vi "ueye check capture status.vi"(8 "error in (no error)":errorcluster, 11 "Camera in":refnum<k24>) -> (0 "error out":errorcluster, 2 "Error List":map{string, u64}(c390), 3 "Camera out":refnum<k24>)   [LabVIEW 2022 SP3, in "Vision.lvlib"]
uses:
  Vision.lvlib
  C:/Users/Caleb/Desktop/nebraska-silicon-lab/pixel-gantry-control/Gantry/Shared Components/bin/uEyeDotNet.dll
  bin/uEyeDotNet.dll
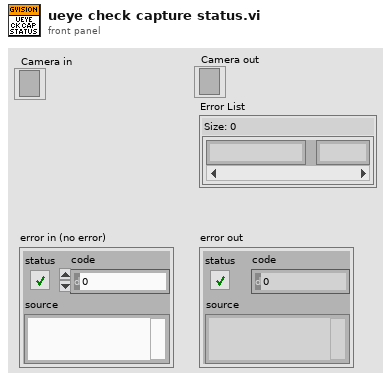
[diagram p1: front panel]
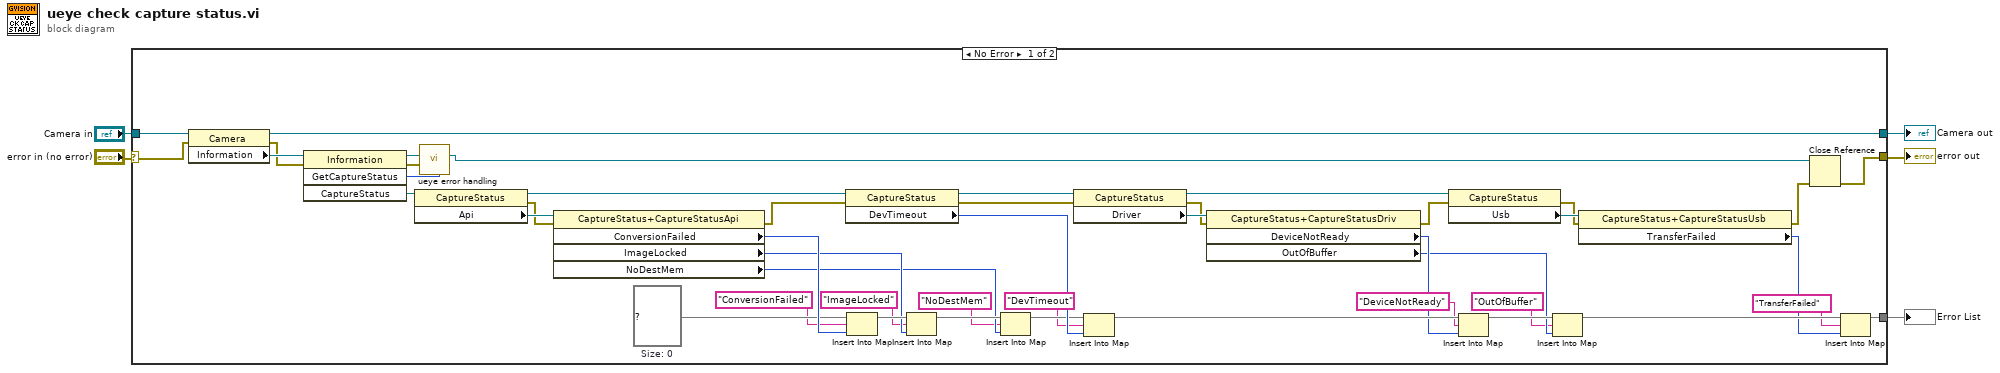
[diagram p0: block diagram]
diagram:
  n1 = case shown="No Error" "error in (no error)" {
    selector: "error in (no error)" -> [w49 w51]
    tunnel: [w6 w51] -> w5
    tunnel: [w7 w52] -> w4
    tunnel: "Camera in" -> [w50 w52]
    tunnel: [w8 _] -> w1
    frame No Error {
      w41 = map{string, u64} {}  # Size: 0
      n2 = property class="Camera"(reference=w50, error in=w49) -> (reference out=w7:refnum<k24>, error out=w47:errorcluster, "Information"=w48:refnum<k24>)
      n3 = invoke class="Information" method="GetCaptureStatus"(reference=w48, error in=w47) -> (reference out=w10:refnum<k24>, error out=w46:errorcluster, "GetCaptureStatus"=w45:i32, "CaptureStatus"=w44:refnum<k24>)  [unwired: 2 in]
      n4 = property class="CaptureStatus"(reference=w44) -> (reference out=w32:refnum<k24>, error out=w33:errorcluster, "Api"=w43:refnum<k24>)  [unwired: 1 in]
      n5 = call "ueye error handling.vi"("Error Code"=w45, "reference in"=w10, "Error In"=w46) -> ()  [unwired: 8 in, 1 out]
      n6 = property class="CaptureStatus+CaptureStatusApi"(reference=w43, error in=w33) -> (error out=w31:errorcluster, "ConversionFailed"=w42:u64, "ImageLocked"=w37:u64, "NoDestMem"=w35:u64)  [unwired: 1 out]
      n7 = property class="CaptureStatus"(reference=w32, error in=w31) -> (reference out=w27:refnum<k24>, error out=w26:errorcluster, "DevTimeout"=w30:u64)
      n8 = Insert Into Map(map in=w41, key="ConversionFailed", value=w42) -> (map out=w39:map{string, u64})  [unwired: 2 out]
      n9 = Insert Into Map(map in=w39, key="ImageLocked", value=w37) -> (map out=w38:map{string, u64})  [unwired: 2 out]
      n10 = Insert Into Map(map in=w38, key="NoDestMem", value=w35) -> (map out=w29:map{string, u64})  [unwired: 2 out]
      n11 = property class="CaptureStatus"(reference=w27, error in=w26) -> (reference out=w17:refnum<k24>, error out=w24:errorcluster, "Driver"=w25:refnum<k24>)
      n12 = Insert Into Map(map in=w29, key="DevTimeout", value=w30) -> (map out=w23:map{string, u64})  [unwired: 2 out]
      n13 = property class="CaptureStatus+CaptureStatusDriv"(reference=w25, error in=w24) -> (error out=w15:errorcluster, "DeviceNotReady"=w22:u64, "OutOfBuffer"=w19:u64)  [unwired: 1 out]
      n14 = property class="CaptureStatus"(reference=w17, error in=w15) -> (error out=w11:errorcluster, "Usb"=w16:refnum<k24>)  [unwired: 1 out]
      n15 = Insert Into Map(map in=w23, key="DeviceNotReady", value=w22) -> (map out=w20:map{string, u64})  [unwired: 2 out]
      n16 = Insert Into Map(map in=w20, key="OutOfBuffer", value=w19) -> (map out=w14:map{string, u64})  [unwired: 2 out]
      n17 = property class="CaptureStatus+CaptureStatusUsb"(reference=w16, error in=w11) -> (error out=w9:errorcluster, "TransferFailed"=w13:u64)  [unwired: 1 out]
      n18 = Close Reference(reference=w10, error in (no error)=w9) -> (error out=w6:errorcluster)
      n19 = Insert Into Map(map in=w14, key="TransferFailed", value=w13) -> (map out=w8:map{string, u64})  [unwired: 2 out]
    }
    frame Error {
    }
  }
  "error out" <- w5
  "Camera out" <- w4
  "Error List" <- w1
